vi "test_set_inline_table_item.vi"() -> ()   [LabVIEW 2020]
uses:
  Table/Table.lvclass
  Doc/Doc.lvclass
  Item/Item.lvclass
  InlineTable/InlineTable.lvclass
panel:
  in  "error in (no error)":errorcluster
  out "removed?":bool
  out "error out":errorcluster
  out "toml_string":string
  in  "toml":string="[vipm.dependencies]\noglib_array = {version = \"1.2.3\"}"
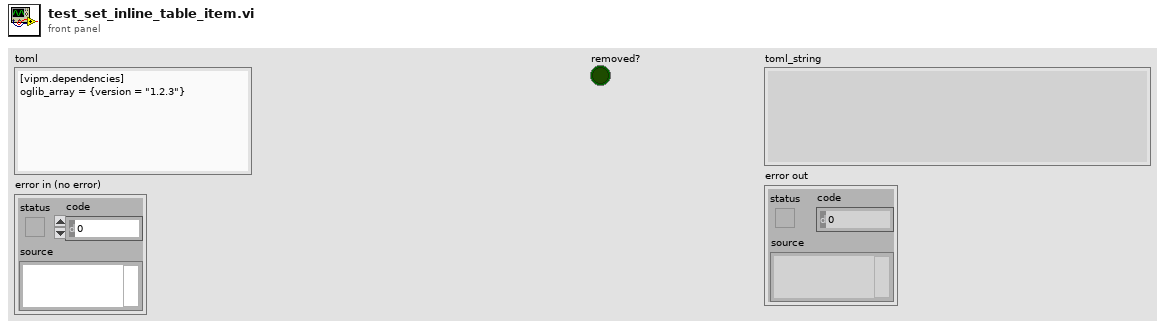
[diagram p1: front panel]
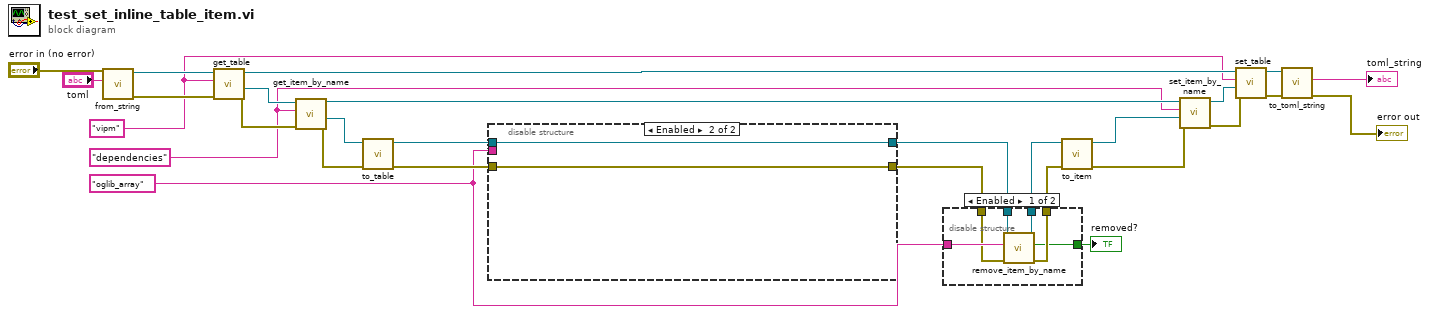
[diagram p0: block diagram]
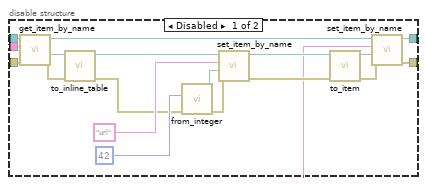
[diagram p2: hidden frame]
diagram:
  w18 = "dependencies" ("table_name")
  w16 = "vipm" ("table_name")
  w8 = "oglib_array" ("item_name")
  n1 = call "from_string.vi"("error in (no error)"="error in (no error)", "toml"="toml") -> ("error out"=w24:errorcluster, "Doc out"=w25:refnum<class "Doc.lvclass">)  [unwired: 8 in]
  n2 = call "get_table.vi"("error in (no error)"=w24, "table_name"=w16, "Doc in"=w25) -> ("error out"=w22:errorcluster, "Table"=w23:refnum<class "Table.lvclass">, "Doc out"=w17:refnum<class "Doc.lvclass">)  [unwired: 6 in]
  n3 = call "get_item_by_name.vi"("error in (no error)"=w22, "item_name"=w18, "Table in"=w23) -> ("error out"=w28:errorcluster, "Item"=w27:refnum<class "Item.lvclass">, "Table out"=w19:refnum<class "Table.lvclass">)  [unwired: 6 in]
  n4 = call "to_table.vi"("error in (no error)"=w28, "Item in"=w27) -> ("error out"=w20:errorcluster, "Table"=w21:refnum<class "Table.lvclass">)  [unwired: 8 in]
  n5 = disable-structure shown="Enabled" {
    disable-tunnel: w21 -> [w46 w48]
    disable-tunnel: w20 -> [w45 w47]
    disable-tunnel: w8 -> [w36 _]
    disable-tunnel: [w35 w48] -> w7
    disable-tunnel: [w34 w47] -> w5
    frame Disabled {
      n6 = call "get_item_by_name.vi"("error in (no error)"=w45, "item_name"=w36, "Table in"=w46) -> ("error out"=w30:errorcluster, "Item"=w33:refnum<class "Item.lvclass">, "Table out"=w40:refnum<class "Table.lvclass">)  [unwired: 6 in]
      n7 = call "to_inline_table.vi"("error in (no error)"=w30, "Item in"=w33) -> ("error out"=w31:errorcluster, "InlineTable"=w32:refnum<class "InlineTable.lvclass">)  [unwired: 8 in]
      n8 = call "from_integer.vi"("error in (no error)"=w31, "value"=i64 42) -> ("error out"=w41:errorcluster, "Item out"=w43:refnum<class "Item.lvclass">)  [unwired: 8 in]
      n9 = call "set_item_by_name.vi"("error in"=w41, "Item"=w43, "key_name"="url", "Table in"=w32) -> ("error out"=w39:errorcluster, "Table out"=w38:refnum<class "InlineTable.lvclass">)  [unwired: 6 in]
      n10 = call "to_item.vi"("error in (no error)"=w39, "Table in"=w38) -> ("error out"=w37:errorcluster, "Item out"=w29:refnum<class "Item.lvclass">)  [unwired: 8 in]
      n11 = call "set_item_by_name.vi"("error in (no error)"=w37, "Item"=w29, "item_name"=w36, "Table in"=w40) -> ("error out"=w34:errorcluster, "Table out"=w35:refnum<class "Table.lvclass">)  [unwired: 6 in]
    }
    frame Enabled {
    }
  }
  n12 = disable-structure shown="Enabled" {
    disable-tunnel: w8 -> [w54 _]
    disable-tunnel: w7 -> [w53 w56]
    disable-tunnel: [w52 w56] -> w6
    disable-tunnel: w5 -> [w51 w55]
    disable-tunnel: [w50 w55] -> w4
    disable-tunnel: [w49 _] -> w3
    frame Enabled {
      n13 = call "remove_item_by_name.vi"("error in (no error)"=w51, "item_name"=w54, "Table in"=w53) -> ("error out"=w50:errorcluster, "removed?"=w49:bool, "Table out"=w52:refnum<class "Table.lvclass">)  [unwired: 6 in]
    }
    frame Disabled {
    }
  }
  "removed?" <- w3
  n14 = call "to_item.vi"("error in (no error)"=w4, "Table in"=w6) -> ("error out"=w13:errorcluster, "Item out"=w1:refnum<class "Item.lvclass">)  [unwired: 8 in]
  n15 = call "set_item_by_name.vi"("error in (no error)"=w13, "Item"=w1, "item_name"=w18, "Table in"=w19) -> ("error out"=w14:errorcluster, "Table out"=w15:refnum<class "Table.lvclass">)  [unwired: 6 in]
  n16 = call "set_table.vi"("error in (no error)"=w14, "Table"=w15, "table_name"=w16, "Doc in"=w17) -> ("error out"=w12:errorcluster, "Doc out"=w11:refnum<class "Doc.lvclass">)  [unwired: 6 in]
  n17 = call "to_toml_string.vi"("error in (no error)"=w12, "Doc in"=w11) -> ("error out"=→"error out":errorcluster, "toml_string"=→"toml_string":string)  [unwired: 7 in, 1 out]
